vi "physicalSettings.vi"() -> ()   [LabVIEW 2020]
panel:
  in  "说明":string
  in  "Lamda 6:":sgl
  in  "Lamda 5:":sgl
  in  "Lamda 4:":sgl
  in  "Lamda 3:":sgl
  in  "Lamda 2:":sgl
  in  "βeff 6:":sgl
  in  "βeff 5:":sgl
  in  "βeff 4:":sgl
  in  "βeff 3:":sgl
  in  "βeff 2:":sgl
  in  "取消":bool caption="Cancel Button"
  in  "确定":bool
  in  "Lamda 1:":sgl
  in  "βeff 1:":sgl
  in  "源强:":sgl
  in  "中子寿命:":sgl
  # "物理参数"
  # "说明"
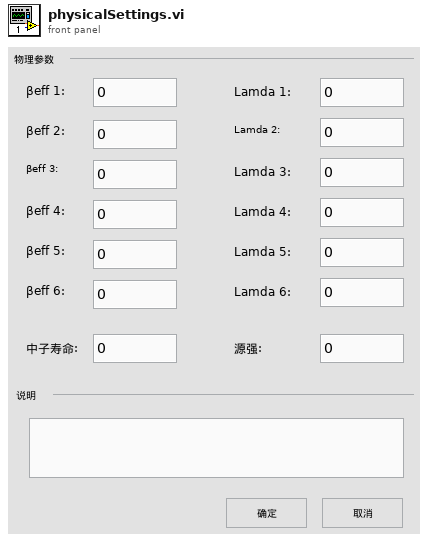
[diagram p1: front panel]
types:
  T1 = enum16{"open", "replace", "create", "open or create", "replace or create", "replace or create with confirmation"}
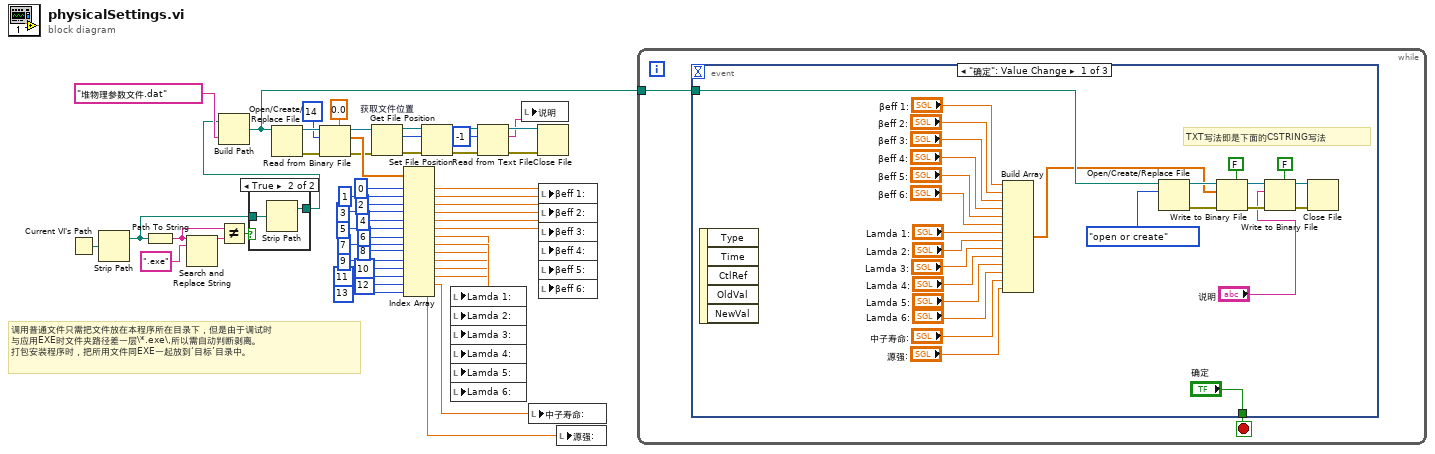
[diagram p0: block diagram]
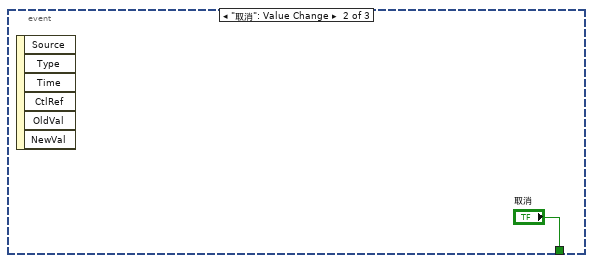
[diagram p3: hidden frame]
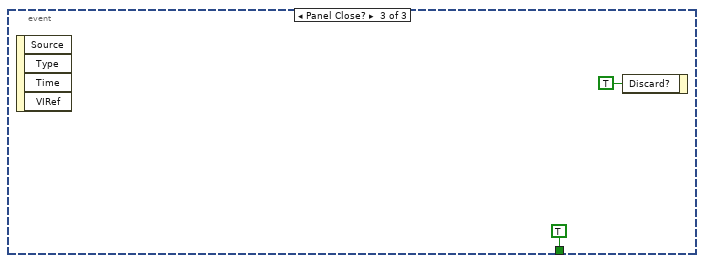
[diagram p4: hidden frame]
diagram:
  # "调用普通文件只需把文件放在本程序所在目录下，但是由于调试时\n与应用EXE时文件夹路径差一层\\*.exe\\,所以需自动判断剥离。\n打包安装程序时，把所用文件同EXE一起放到‘目标’目录中。"
  n1 = Current VI's Path() -> (path=w23:path)
  n2 = Strip Path(path=w23) -> (stripped path=w18:path)  [unwired: 1 out]
  n3 = Path To String(path=w18) -> (string=w20:string)
  n4 = Search and Replace String(input string=w20, search string=".exe" ("搜索字符串")) -> (result string=w21:string)  [unwired: 6 in, 3 out]
  n5 = Not Equal?(x=w20, y=w21) -> (x != y?=w19:bool)
  n6 = case shown="True" w19 {
    tunnel: w18 -> [w54 w56]
    tunnel: [w54 w55] -> w17
    frame False {
    }
    frame True {
      n7 = Strip Path(path=w56) -> (stripped path=w55:path)  [unwired: 1 out]
    }
  }
  n8 = Build Path(base path=w17, name or relative path="堆物理参数文件.dat") -> (appended path=w31:path)
  n9 = Open/Create/Replace File(file path (use dialog)=w31) -> (refnum out=w39:refnum<file>, error out=w38:errorcluster)  [unwired: 5 in, 1 out]
  n10 = Read from Binary File(5:sgl 0.0 ("byte stream type"), 8:w38, 10:14 ("count"), 11:w39) -> (0:w29:errorcluster, 2:w35:sgl[], 3:w30:refnum<file>)  [unwired: 2 in, 1 out]
  n11 = Get File Position "获取文件位置"(4:w29, 7:w30) -> (0:w33:errorcluster, 2:w28:i64, 3:w34:refnum<file>)
  n12 = Index Array(array=w35, index #1=0, index #2=1, index #3=2, index #4=3, index #5=4, index #6=5, index #7=6, index #8=7, index #9=8, index #10=9, index #11=10, index #12=11, index #13=12, index #14=13) -> (element #1=w14:sgl, element #2=w13:sgl, element #3=w12:sgl, element #4=w9:sgl, element #5=w8:sgl, element #6=w7:sgl, element #7=w15:sgl, element #8=w16:sgl, element #9=w11:sgl, element #10=w10:sgl, element #11=w6:sgl, element #12=w5:sgl, element #13=w4:sgl, element #14=w3:sgl)
  n13 = Set File Position(offset (in bytes) (0)=w28, refnum=w34, error in=w33) -> (refnum out=w27:refnum<file>, error out=w26:errorcluster)  [unwired: 1 in]
  n14 = local write "Lamda 1:"(w15) -> ()
  n15 = local write "Lamda 2:"(w16) -> ()
  n16 = local write "Lamda 3:"(w11) -> ()
  n17 = local write "Lamda 4:"(w10) -> ()
  n18 = local write "Lamda 5:"(w6) -> ()
  n19 = local write "Lamda 6:"(w5) -> ()
  n20 = Read from Text File(file (use dialog)=w27, count=-1, error in=w26) -> (refnum out=w25:refnum<file>, text=w1:string, error out=w24:errorcluster)  [unwired: 2 out]
  n21 = local write "说明"(w1) -> ()
  n22 = local write "中子寿命:"(w4) -> ()
  n23 = Close File(refnum=w25, error in=w24) -> ()  [unwired: 2 out]
  n24 = local write "βeff 1:"(w14) -> ()
  n25 = local write "βeff 2:"(w13) -> ()
  n26 = local write "βeff 3:"(w12) -> ()
  n27 = local write "βeff 4:"(w9) -> ()
  n28 = local write "βeff 5:"(w8) -> ()
  n29 = local write "βeff 6:"(w7) -> ()
  n30 = local write "源强:"(w3) -> ()
  n31 = while {
    tunnel: w31 -> [w57]
    stop <- w58 stop-if-true
    n32 = event shown="[0] \"确定\": Value Change" {
      selector: _ -> [_ _ _]
      dyn-events: _ -> [_ _ _]
      timeout: _ -> [_ _ _]
      tunnel: ["确定" "取消" TRUE ("取消")] -> w58
      tunnel: w57 -> [w75 _ _]
      event "确定": Value Change {
        # "TXT写法即是下面的CSTRING写法"
        n33 = event-data() -> ()  [unwired: 1 in, 5 out]
        n34 = Build Array("βeff 1:", "βeff 2:", "βeff 3:", "βeff 4:", "βeff 5:", "βeff 6:", "Lamda 1:", "Lamda 2:", "Lamda 3:", "Lamda 4:", "Lamda 5:", "Lamda 6:", "中子寿命:", "源强:") -> (w61:sgl[])
        n35 = Open/Create/Replace File(file path (use dialog)=w75, operation (0:open)=T1."open or create" ("操作(0:open)")) -> (refnum out=w74:refnum<file>, error out=w73:errorcluster)  [unwired: 4 in, 1 out]
        n36 = Write to Binary File(file (use dialog)=w74, data=w61, error in=w73, 5:FALSE ("预置数组或字符串大小？(T)")) -> (refnum out=w64:refnum<file>, error out=w63:errorcluster)  [unwired: 2 in, 1 out]
        n37 = Write to Binary File(file (use dialog)=w64, data="说明", error in=w63, 5:FALSE ("预置数组或字符串大小？(T)")) -> (refnum out=w66:refnum<file>, error out=w65:errorcluster)  [unwired: 2 in, 1 out]
        n38 = Close File(refnum=w66, error in=w65) -> ()  [unwired: 2 out]
      }
      event "取消": Value Change {
        n39 = event-data() -> ()  [unwired: 1 in, 6 out]
      }
      event Panel Close? {
        n40 = event-data() -> ()  [unwired: 1 in, 4 out]
        n41 = event-data("Discard?"=TRUE) -> ()  [unwired: 1 in, 1 out]
      }
    }
  }
